vi "Init_Tracks&Coord-2.vi"() -> (0 "[OUT] Tracks, Coordinates":T1)   [LabVIEW 2013]
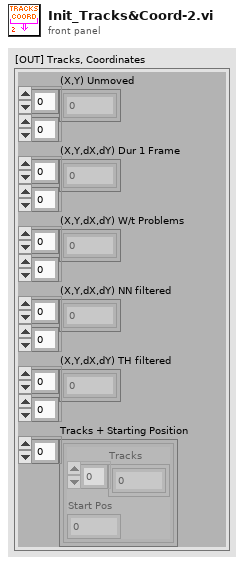
[diagram p1: front panel]
types:
  T1 = cluster{"(X,Y) Unmoved":dbl[][], "(X,Y,dX,dY) Dur 1 Frame":dbl[][], "(X,Y,dX,dY) W/t Problems":dbl[][], "(X,Y,dX,dY) NN filtered":dbl[][], "(X,Y,dX,dY) TH filtered":dbl[][], "Tracks + Starting Position":cluster{"Tracks":dbl[], "Start Pos":i32}[]}
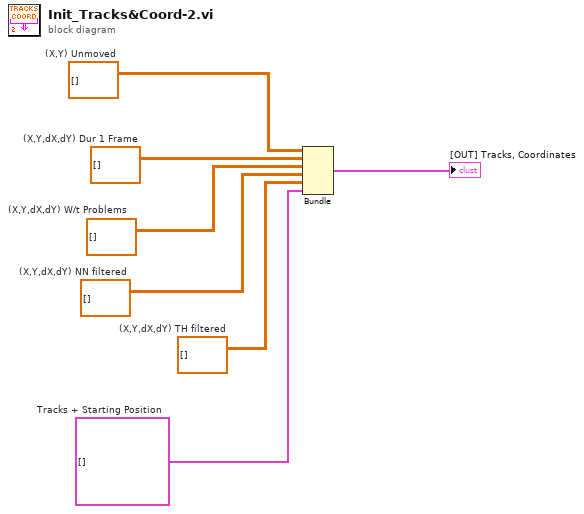
[diagram p0: block diagram]
diagram:
  w2 = cluster{"Tracks":dbl[], "Start Pos":i32}[] []  # Tracks + Starting Position
  w4 = dbl[][] []  # (X,Y,dX,dY) TH filtered
  w3 = dbl[][] []  # (X,Y,dX,dY) NN filtered
  w6 = dbl[][] []  # (X,Y,dX,dY) Dur 1 Frame
  w7 = dbl[][] []  # (X,Y) Unmoved
  w5 = dbl[][] []  # (X,Y,dX,dY) W/t Problems
  n1 = Bundle("(X,Y) Unmoved"=w7, "(X,Y,dX,dY) Dur 1 Frame"=w6, "(X,Y,dX,dY) W/t Problems"=w5, "(X,Y,dX,dY) NN filtered"=w3, "(X,Y,dX,dY) TH filtered"=w4, "Tracks + Starting Position"=w2) -> (→"[OUT] Tracks, Coordinates":T1)  [unwired: 1 in]
